vi "GetParam.vi"(8 "error in (no error)":errorcluster caption="entrée d'erreur (pas d'erreur)", 11 "20newsgroups_vectorized.lvclass":refnum<class "20newsgroups_vectorized.lvclass">) -> (0 "error out":errorcluster caption="sortie d'erreur", 2 "fetch_20newsgroups_vectorized":T1={"subset"="train", "remove"=[], "download_if_missing"=TRUE, "normalize"=TRUE, "Returns"="Data"}, 3 "20newsgroups_vectorized.lvclass 2":refnum<class "20newsgroups_vectorized.lvclass">)   [LabVIEW 2020, in "20newsgroups_vectorized.lvclass"]
doc: "Get parameters"
uses:
  20newsgroups_vectorized.lvclass
  20newsgroups_vectorized.lvclass/20newsgroups_vectorized.ctl
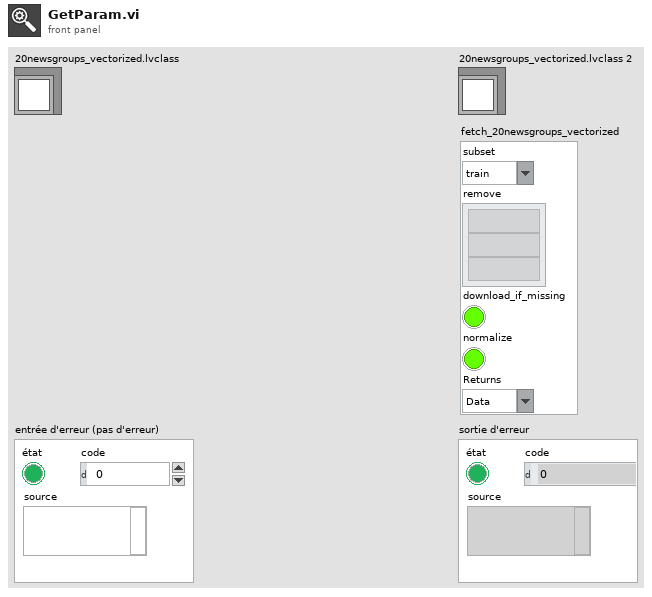
[diagram p1: front panel]
types:
  T1 = cluster{"subset":string, "remove":string[], "download_if_missing":bool, "normalize":bool, "Returns":string}
  T2 = cluster{"subset":string, "remove":string[], " download_if_missing ":bool, "normalize":bool, "Returns":string}
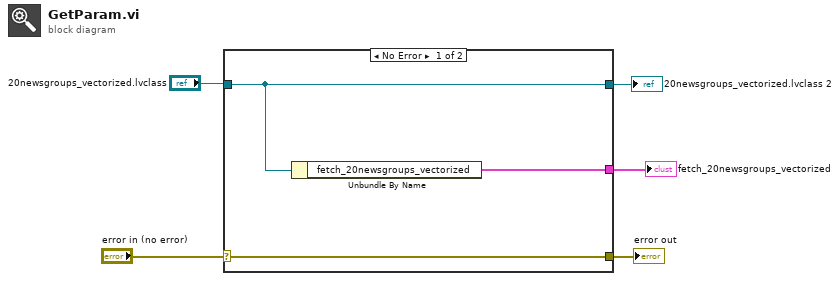
[diagram p0: block diagram]
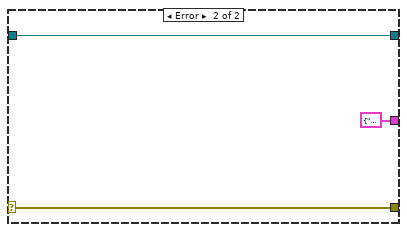
[diagram p2: hidden frame]
diagram:
  n1 = case shown="No Error" "error in (no error)" {
    selector: "error in (no error)" -> [w8 w10]
    tunnel: [w8 w10] -> w4
    tunnel: [w7 w11] -> w2
    tunnel: "20newsgroups_vectorized.lvclass" -> [w7 w11]
    tunnel: [w6 T2 {"subset"="", "remove"=[], " download_if_missing "=FALSE, "normalize"=FALSE, "Returns"=""} ("fetch_20newsgroups_vectorized")] -> w1
    frame No Error {
      n2 = Unbundle By Name(w7) -> ("fetch_20newsgroups_vectorized"=w6:T2)
    }
    frame Error {
    }
  }
  "error out" <- w4
  "fetch_20newsgroups_vectorized" <- w1
  "20newsgroups_vectorized.lvclass 2" <- w2
